vi "Draw Legend Cluster.vi"(8 "error in (no error)":errorcluster, 9 "Plot Area Ref":refnum<vi>, 10 "Number Of Rows":i32, 11 "2D Compass.lvclass in":refnum<class "2D Compass.lvclass">) -> (0 "error out":errorcluster, 1 "Legend Cluster":T1(array[cluster]), 3 "2D Compass.lvclass out":refnum<class "2D Compass.lvclass">)   [LabVIEW 2020, in "2D Compass.lvclass"]
uses:
  <vilib>/Math Plots/2D Math Plots/2D Compass/2D Compass/2D Compass.lvclass
  <vilib>/Math Plots/2D Math Plots/2D Compass/2D Compass/2D Compass.lvclass/2D Compass.ctl
  <vilib>/Math Plots/2D Math Plots/2D Plot/2D Plot/2D Plot.lvclass
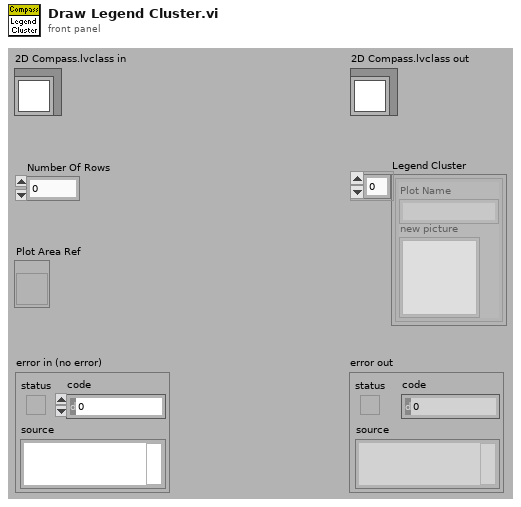
[diagram p1: front panel]
types:
  T1 = cluster{"Plot Name":string, "new picture":picture}[]
  T2 = typedef "2D Plot.lvclass/Plot Property Array.ctl" = T3[]
  T3 = typedef "2D Plot.lvclass/Plot Property.ctl" = cluster{"Bar Plot Style":u8, "DigitalLineStyle":u8, "TransitionLocation":u8, "Transition Type":u8, "Fill To":i16, "Fill/Pt. Color":u32, "Label Style":u8, "Line Style":u8, "Line Width":u8, "Plot Color":u32, "Plot Interpolation":u8, "Plot Name":string, "Point Style":u8, "Visible?":bool, "XScaleIdx":u32, "YScaleIdx":u32}
  T4 = cluster{"Width":u16, "Style":enum32{"Solid", "Dash", "Dot", "DashDot", "DashDotDot"}}
  T5 = cluster{"left":i16, "top":i16, "right":i16, "bottom":i16}
  T6 = cluster{"Plot Name":string, "new picture":picture}
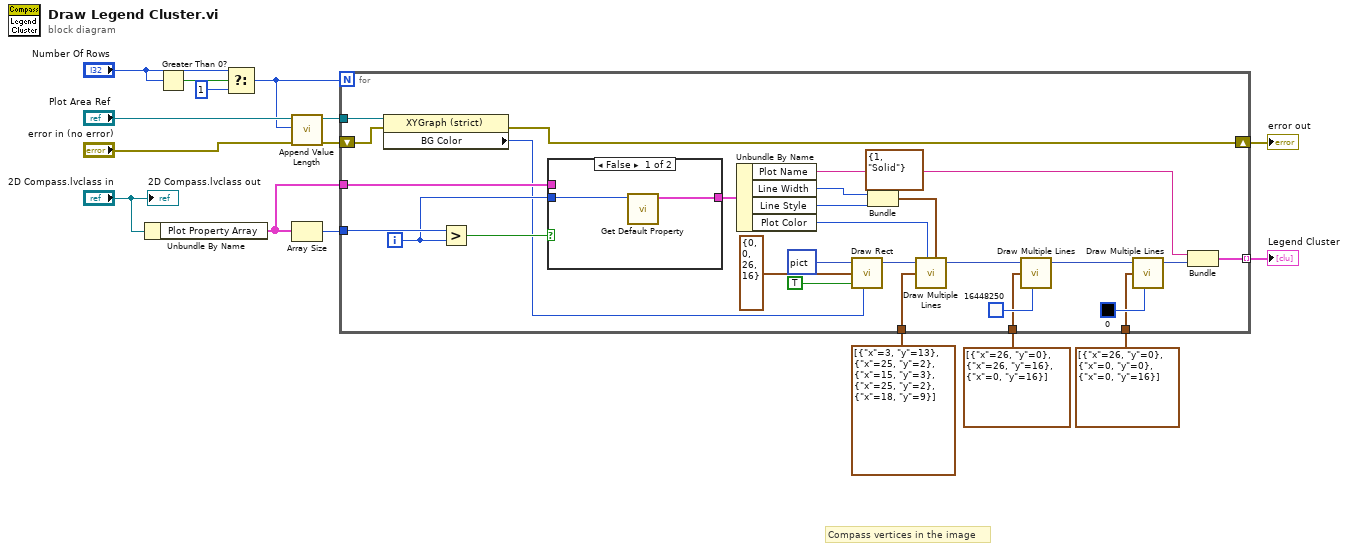
[diagram p0: block diagram]
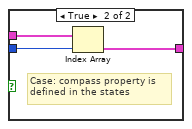
[diagram p2: hidden frame]
diagram:
  # "Compass vertices in the image"
  n1 = Unbundle By Name("2D Compass.lvclass in") -> ("Plot Property Array"=w12:T2)
  n2 = Greater Than 0?(x="Number Of Rows") -> (x > 0?=w16:bool)
  n3 = Select(t="Number Of Rows", s=w16, f=1) -> (s? t:f=w4:i32)
  n4 = call <vilib>:"Append Value Length.vi"("error in (no error)"="error in (no error)", "Expect Value Length"=w4, "Plot Area Ref In"="Plot Area Ref") -> ("error out"=w5:errorcluster, "Plot Area Ref Out"=w7:refnum<vi>)  [unwired: 1 in, 6 out]
  n5 = Array Size(array=w12) -> (size(s)=w14:i32)
  n6 = for {
    N: w4 -> [_]
    tunnel: w12 -> [w34]
    tunnel: [w38] -> w10 mode=indexing
    tunnel: w14 -> [w36]
    tunnel: w7 -> [w29]
    shift-right: [w17] -> w9
    shift-left: w5 -> [w27]
    tunnel: cluster{"x":i16, "y":i16}[] [{"x"=3, "y"=13}, {"x"=25, "y"=2}, {"x"=15, "y"=3}, {"x"=25, "y"=2}, {"x"=18, "y"=9}] ("line endpoints") -> [w20]
    tunnel: cluster{"x":i16, "y":i16}[] [{"x"=26, "y"=0}, {"x"=26, "y"=16}, {"x"=0, "y"=16}] ("line endpoints") -> [w19]
    tunnel: cluster{"x":i16, "y":i16}[] [{"x"=26, "y"=0}, {"x"=0, "y"=0}, {"x"=0, "y"=16}] ("line endpoints") -> [w18]
    i -> [w33]
    n7 = property class="XYGraph (strict)"(reference=w29, error in=w27) -> (error out=w17:errorcluster, "BG Color"=w28:u32)  [unwired: 1 out]
    n8 = Greater?(x=w36, y=w33) -> (0:w35:bool)
    n9 = case shown="False" w35 {
      tunnel: w34 -> [_ w49]
      tunnel: w33 -> [w46 w48]
      tunnel: [w45 w47] -> w32
      frame False {
        n10 = call <vilib>:"Get Default Property.vi"("Index"=w46) -> ("Temporary Property"=w45:T3)  [unwired: 3 in, 7 out]
      }
      frame True {
        # "Case: compass property is \ndefined in the states"
        n11 = Index Array(array=w49, index=w48) -> (element=w47:T3)
      }
    }
    n12 = Unbundle By Name(w32) -> ("Plot Name"=w39:string, "Line Width"=w42:u8, "Line Style"=w41:u8, "Plot Color"=w31:u32)
    n13 = call <vilib>:"Draw Rect.vi"("picture"=picture data[5B], "rect"=T5 {"left"=0, "top"=0, "right"=26, "bottom"=16}, "fill?(F)"=TRUE, "color(black)"=w28) -> ("new picture"=w43:picture)  [unwired: 1 in, 4 out]
    n14 = Bundle(cluster=T4 {"Width"=1, "Style"=enum."Solid"} ("pen"), "Width"=w42, "Style"=w41) -> (w30:T4)
    n15 = call <vilib>:"Draw Multiple Lines.vi"("picture"=w43, "line endpoints"=w20, "color(black)"=w31, "pen"=w30) -> ("new picture"=w24:picture)  [unwired: 1 in, 4 out]
    n16 = call <vilib>:"Draw Multiple Lines.vi"("picture"=w24, "line endpoints"=w19, "color(black)"=u32 16448250) -> ("new picture"=w22:picture)  [unwired: 2 in, 4 out]
    n17 = call <vilib>:"Draw Multiple Lines.vi"("picture"=w22, "line endpoints"=w18, "color(black)"=u32 0) -> ("new picture"=w21:picture)  [unwired: 2 in, 4 out]
    n18 = Bundle("Plot Name"=w39, "new picture"=w21) -> (w38:T6)  [unwired: 1 out]
  }
  "Legend Cluster" <- w10
  "error out" <- w9
  "2D Compass.lvclass out" <- "2D Compass.lvclass in"
